vi "OSICS_Set_Wavelength.vi"(7 "OSICS slot":i32=1 min=1 max=8, 8 "error in":errorcluster, 9 "WL/Frequency Value":dbl format="%#.3f", 10 "WL/F unit (False:nm)":bool, 11 "VISA IN":refnum<visa-resource-name>) -> (0 "error out":errorcluster, 3 "VISA OUT":refnum<visa-resource-name>, 5 "ERR":i32)   [LabVIEW 2014, in "OSICS_LIB.lvlib"]
doc: "This Vi sets the Wavelength/Frequency unit and value of OSICS laser modules.\nModules: DFB, SLED, ECL, T100, TLS-50, and TLS-AG."
uses:
  OSICS_LIB.lvlib
panel:
  # "BASIC Function to set wavelength or frequency\nof OSICS Laser Modules"
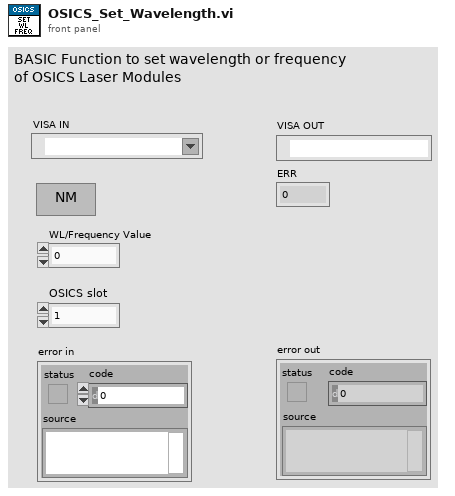
[diagram p1: front panel]
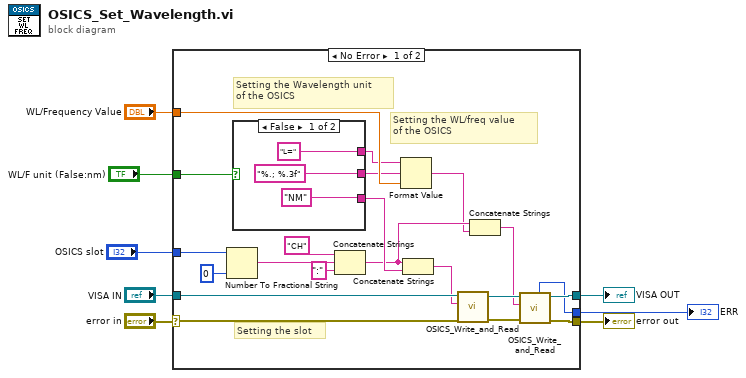
[diagram p0: block diagram]
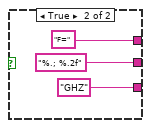
[diagram p2: hidden frame]
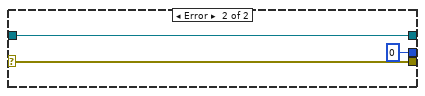
[diagram p3: hidden frame]
diagram:
  n1 = case shown="No Error" "error in" {
    selector: "error in" -> [w15 w37]
    tunnel: "WL/F unit (False:nm)" -> [w29 _]
    tunnel: "VISA IN" -> [w16 w38]
    tunnel: "WL/Frequency Value" -> [w28 _]
    tunnel: [w27 w38] -> w7
    tunnel: [w26 w37] -> w6
    tunnel: [w19 0 ("ERR")] -> w2
    tunnel: "OSICS slot" -> [w24 _]
    frame No Error {
      # "Setting the slot"
      # "Setting the WL/freq value\nof the OSICS"
      # "Setting the Wavelength unit\nof the OSICS"
      n2 = Number To Fractional String(number=w24, precision (6)=i16 0) -> (F-format string=w21:string)  [unwired: 2 in]
      n3 = case shown="False" w29 {
        tunnel: ["%.; %.3f" ("format string") "%.; %.2f" ("format string")] -> w25
        tunnel: ["L=" "F="] -> w12
        tunnel: ["NM" "GHZ"] -> w14
        frame False {
        }
        frame True {
        }
      }
      n4 = Concatenate Strings("CH" ("string"), w21, ":" ("string")) -> (w11:string)
      n5 = Format Value(string ("")=w12, format string=w25, value (0)=w28) -> (output string=w10:string)
      n6 = Concatenate Strings(w11, w14) -> (w13:string)
      n7 = call "OSICS_Write_and_Read.vi"("error in (no error)"=w15, "String to Send"=w13, "VISA IN"=w16) -> ("error out"=w18:errorcluster, "VISA OUT"=w17:refnum<visa-resource-name>)  [unwired: 5 in, 2 out]
      n8 = Concatenate Strings(w11, w10) -> (w9:string)
      n9 = call "OSICS_Write_and_Read.vi"("error in (no error)"=w18, "String to Send"=w9, "VISA IN"=w17) -> ("error out"=w26:errorcluster, "VISA OUT"=w27:refnum<visa-resource-name>, "ERR"=w19:i32)  [unwired: 5 in, 1 out]
    }
    frame Error {
    }
  }
  "error out" <- w6
  "VISA OUT" <- w7
  "ERR" <- w2
